vi "Call Gabor transform (V0.10).vi"(0 "wFormDSP ref in":refnum<class "GSwFormDSP.lvclass">, 5 "error in (no error)":errorcluster, 7 "Application Name":string="GenUtil", 9 "State Queue":string[](array[string])=["SC >>> Initialize"]) -> (19 "error out":errorcluster)   [LabVIEW 2022 SP3, in "SigMath.lvclass"]
uses:
  SigMath.lvclass
  API/GSwFormDSP_class/GSwFormDSP.lvclass
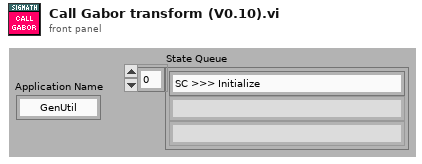
[diagram p1: front panel]
types:
  T1 = typedef "SigMath.lvclass/SigMath Data.ctl" = cluster{"New Time Data Obj?":bool, "GSwFormDSP":refnum<class "GSwFormDSP.lvclass">}
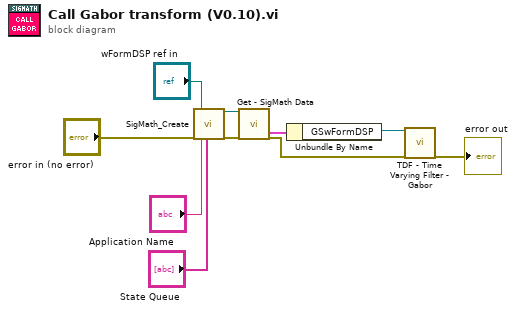
[diagram p0: block diagram]
diagram:
  n1 = call "SigMath_Create.vi"("error in (no error)"="error in (no error)", "Time Data"="wFormDSP ref in", "Application Name"="Application Name", "State Queue"="State Queue") -> ("reference out"=w1:refnum<class "SigMath.lvclass">, "error out"=w3:errorcluster)  [unwired: 14 in]
  n2 = call "Get - SigMath Data.vi"("reference in"=w1, "error in (no error)"=w3) -> ("SigMath Data"=w6:T1, "error out"=w4:errorcluster)  [unwired: 15 in, 1 out]
  n3 = Unbundle By Name(w6) -> ("GSwFormDSP"=w5:refnum<class "GSwFormDSP.lvclass">)
  n4 = call "TDF - Time Varying Filter - Gabor.vi"("reference in"=w5, "error in (no error)"=w4) -> ("error out"=→"error out":errorcluster)  [unwired: 16 in, 1 out]
